vi "Close.vi"(8 "error in (no error)":errorcluster, 11 "Executor":refnum<class "Executor.lvclass">) -> (0 "error out":errorcluster)   [LabVIEW 2014, in "Executor.lvclass"]
uses:
  Executor.lvclass
  Executor.lvclass/Executor.ctl
  Controls/Executor Data - STYP.ctl
  Controls/Executor Status - STYP.ctl
  Controls/Job Results - STYP.ctl
  <vilib>/ActorFramework/Message Enqueuer/Message Enqueuer.lvclass
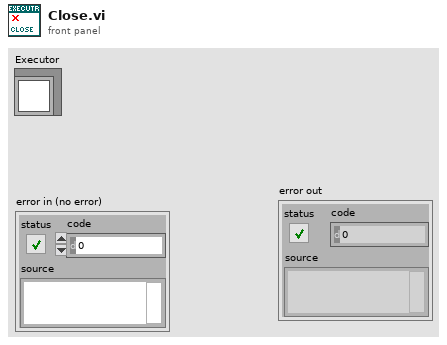
[diagram p1: front panel]
types:
  T1 = typedef "Executor Data - STYP.ctl" = cluster{"Status":T2, "Result Queue":refnum<queue>, "Actor Enquerer":refnum<class "Message Enqueuer.lvclass">}
  T2 = typedef "Executor Status - STYP.ctl" = cluster{"Executor Name":string, "Status":bool}
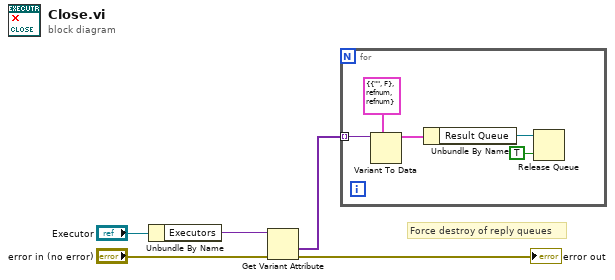
[diagram p0: block diagram]
diagram:
  # "Force destroy of reply queues"
  n1 = Unbundle By Name("Executor") -> ("Executors"=w3:variant)
  n2 = Get Variant Attribute(Variant=w3, error in="error in (no error)") -> (values=w2:variant[], error out=→"error out":errorcluster)  [unwired: 2 in, 2 out]
  n3 = for {
    tunnel: w2 -> [w9] mode=indexing
    n4 = Variant To Data(type=T1 {"Status"={"Executor Name"="", "Status"=FALSE}, "Result Queue"=refnum, "Actor Enquerer"=refnum} ("Executor Data"), Variant=w9) -> (data=w8:T1)  [unwired: 1 in, 1 out]
    n5 = Unbundle By Name(w8) -> ("Result Queue"=w7:refnum<queue>)
    n6 = Release Queue(queue=w7, force destroy? (F)=TRUE) -> ()  [unwired: 1 in, 3 out]
  }
